vi "NovaParts.vi"() -> ()   [LabVIEW 2012]
uses:
  <vilib>/addons/database/Connection.llb/DB Tools Open Connec (Path).vi
  <vilib>/addons/database/Connection.llb/Conn Execute.vi
  <vilib>/addons/database/Recordset.llb/Rec Fetch Recordset Data (R).vi
  <vilib>/addons/database/Recordset.llb/Rec Destroy - Connection.vi
  <vilib>/Utility/file.llb/Write To Spreadsheet File (string).vi
  <vilib>/addons/database/_DB Variant To Data/Database Variant To Data.xnode
  <vilib>/addons/database/NI_Database_API.lvlib
panel:
  out "error out":errorcluster
  out "Array 2":string[][](array[string])
  out "spreadsheet string":string
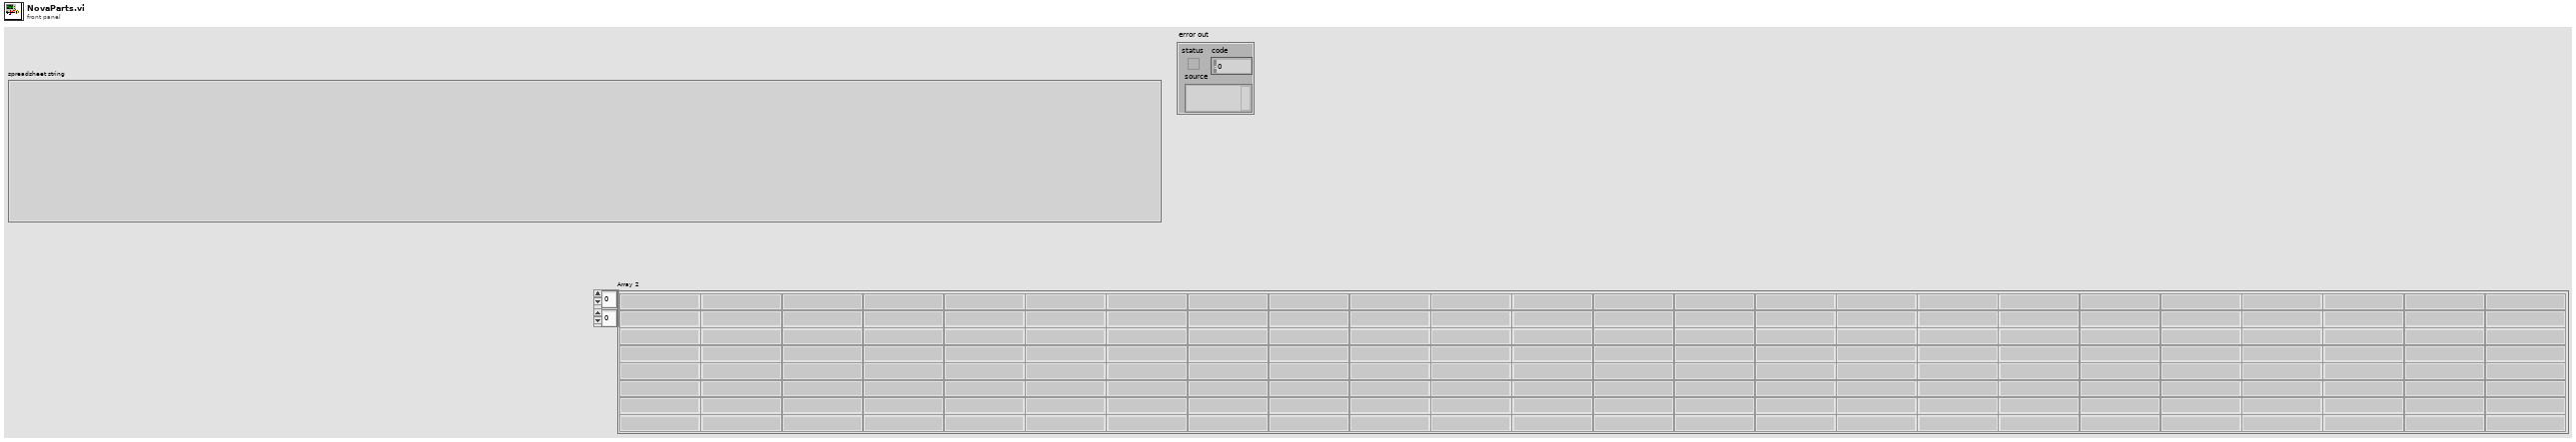
[diagram p1: front panel]
types:
  T1 = typedef "NI_Database_API.lvlib/Conn ObjectReference.ctl" = refnum<k1>
  T2 = typedef "NI_Database_API.lvlib/Rec ObjectReference.ctl" = refnum<k1>
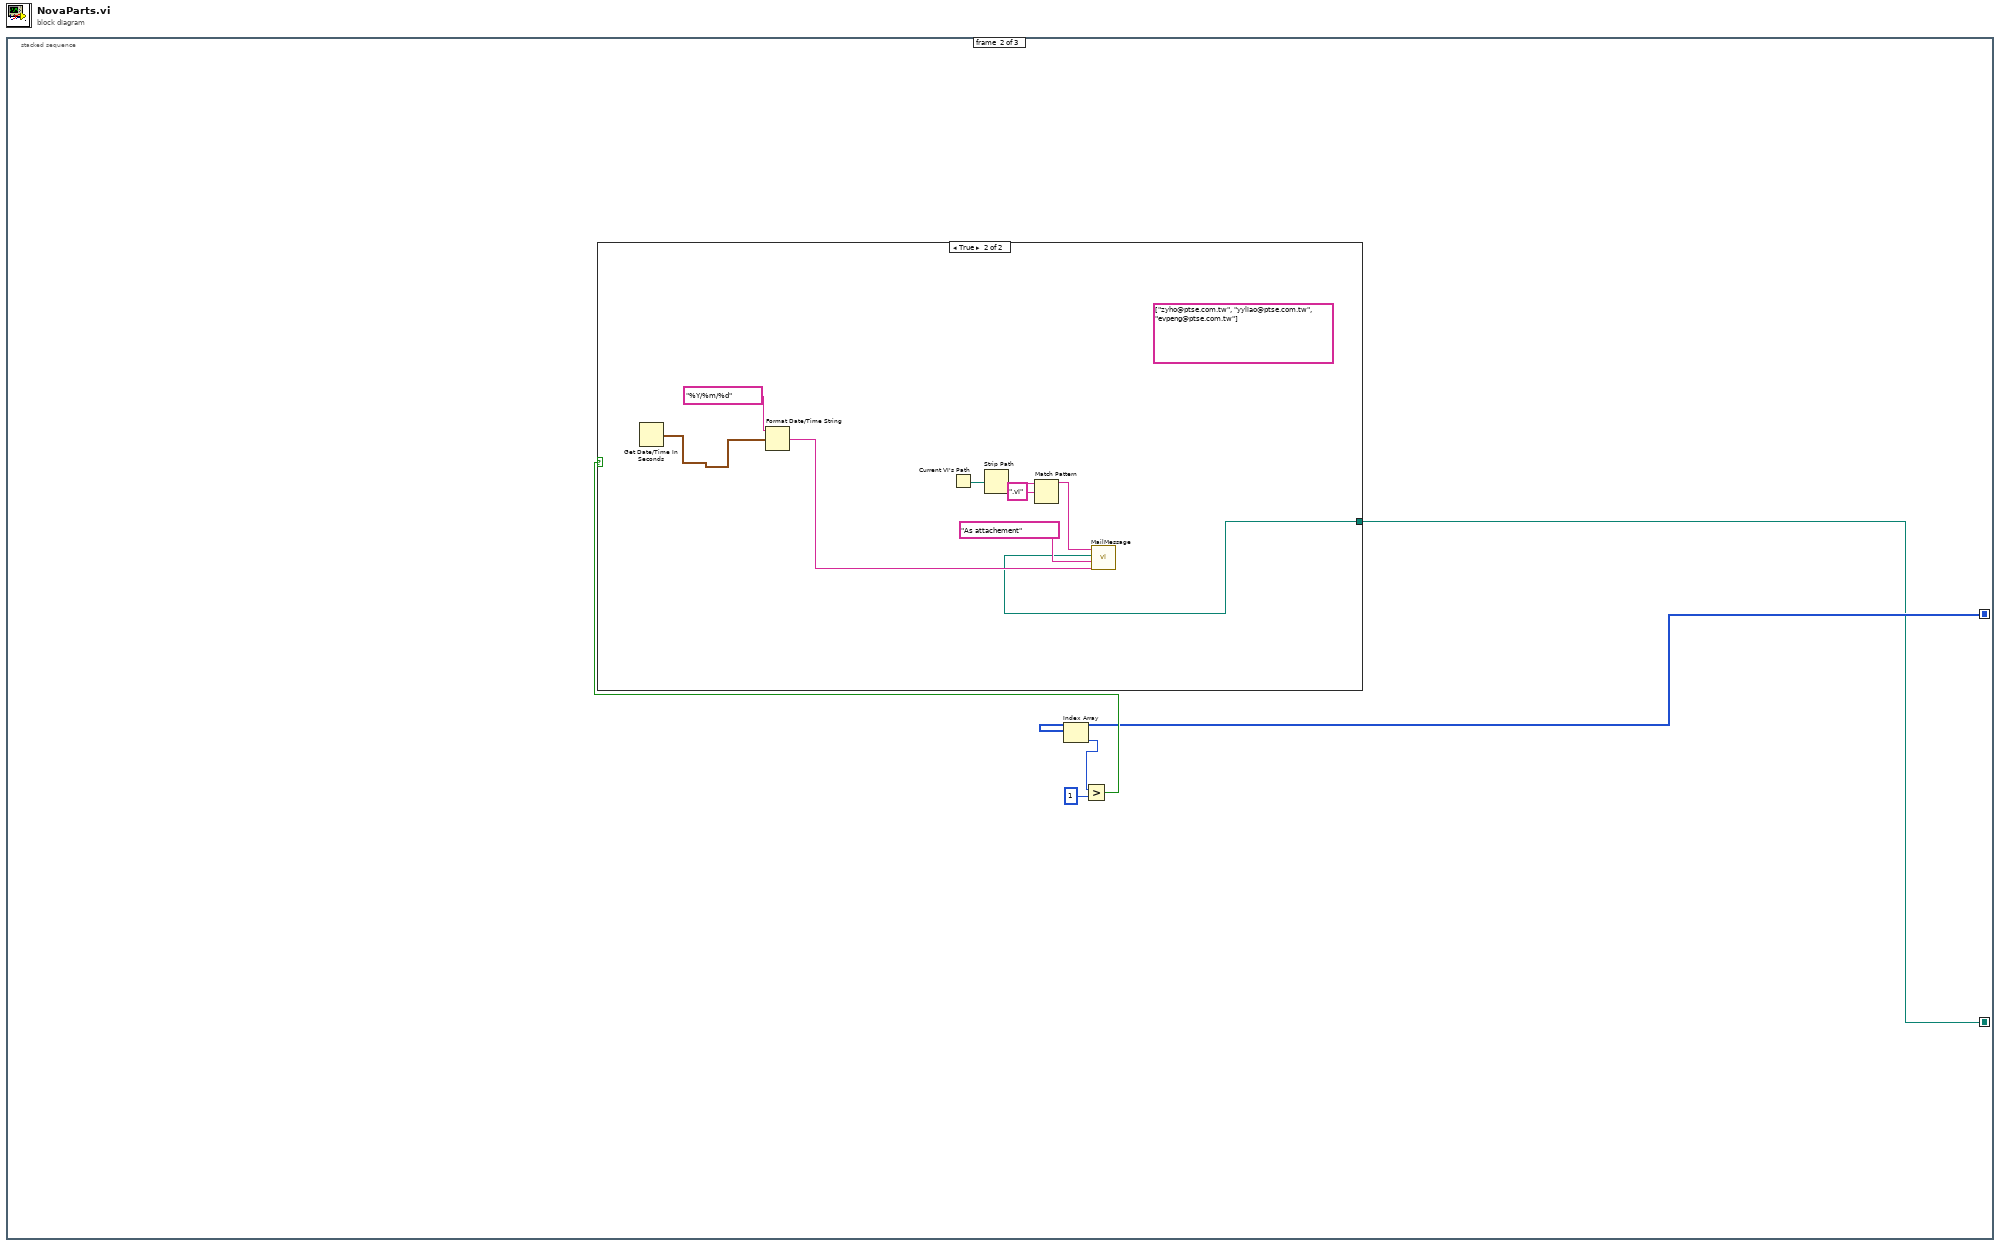
[diagram p0: block diagram]
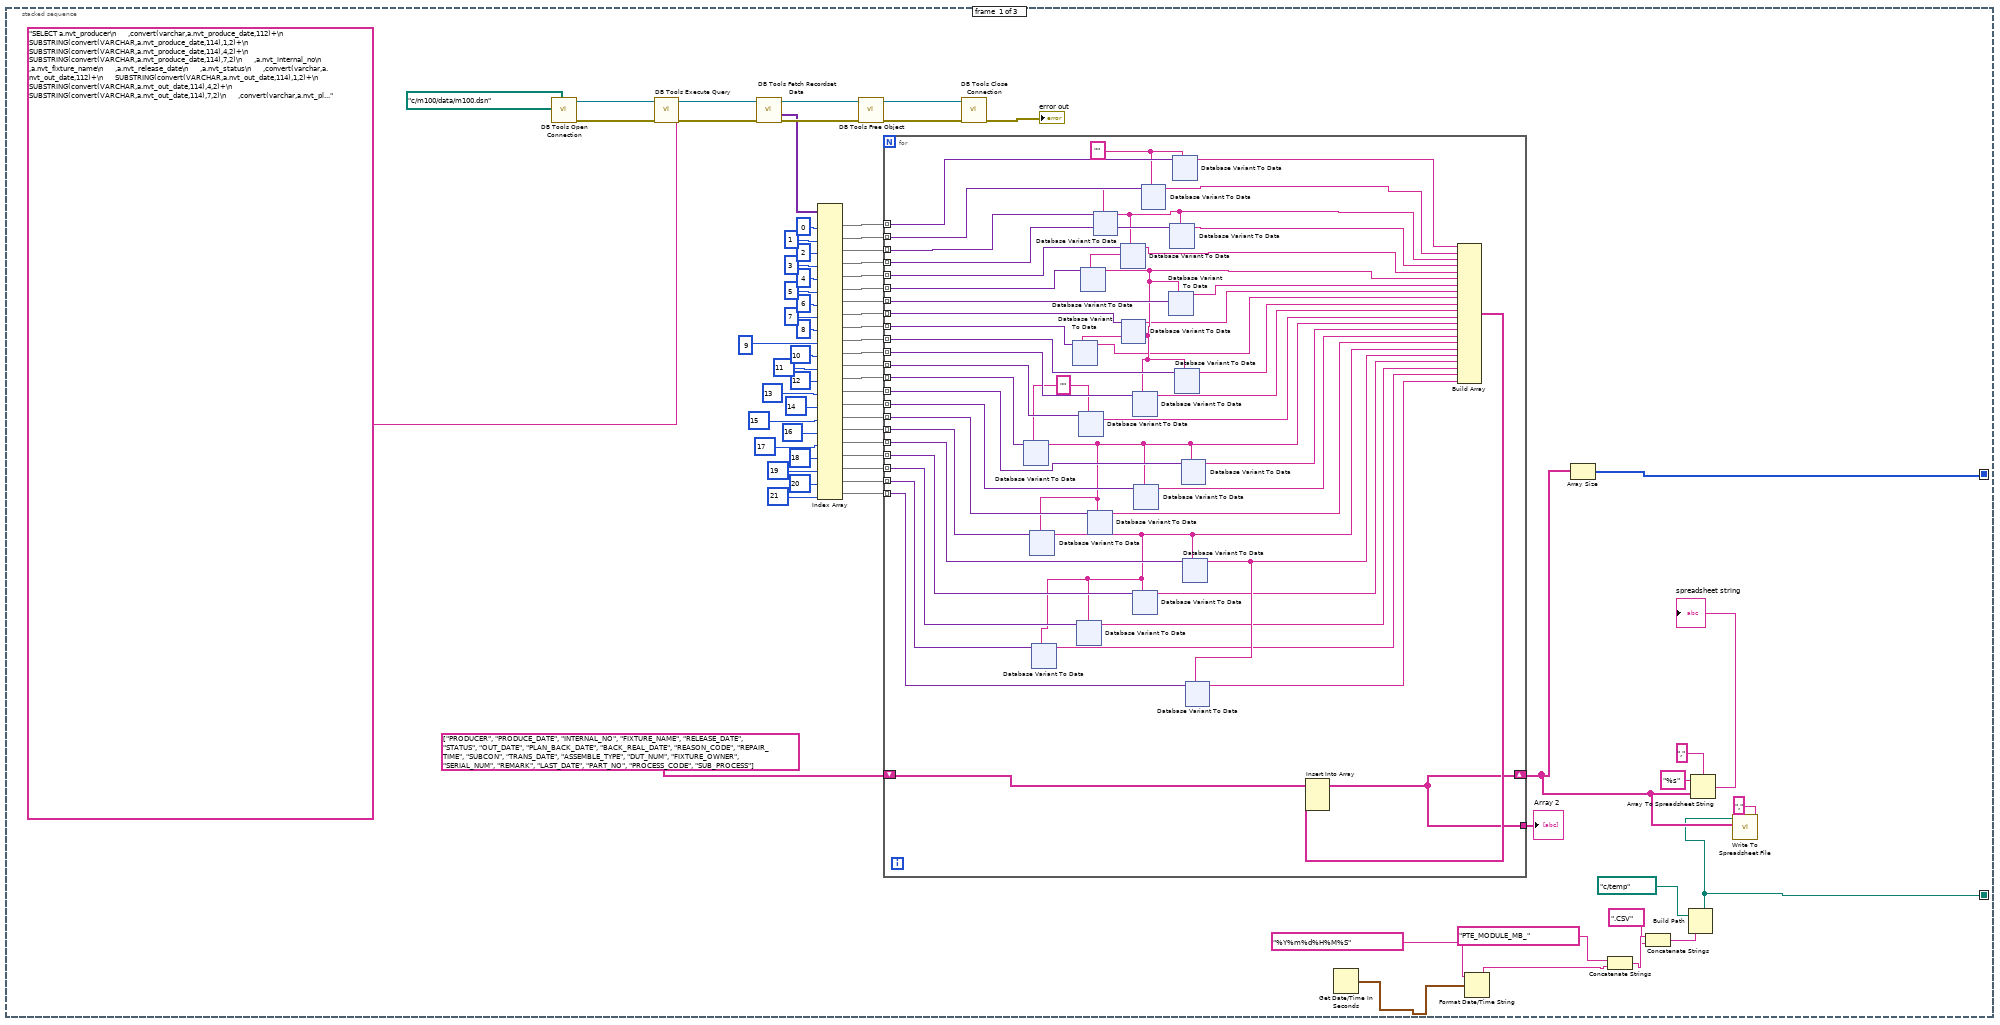
[diagram p2: hidden frame]
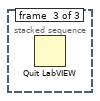
[diagram p4: hidden frame]
diagram:
  n1 = stacked-sequence {
    seq-local: [w41 _ _] -> [_ w828 _]
    seq-local: [w11 _ _] -> [_ w827 _]
    frame #0 {
      n2 = call-poly <vilib>:"DB Tools Open Connection.vi"("connection information"=path "c:/m100/data/m100.dsn") -> ("error out"=w68:errorcluster, "connection reference"=w72:T1)  [unwired: 7 in]
      n3 = call-poly <vilib>:"DB Tools Execute Query.vi"("error in (no error)"=w68, "SQL query"="SELECT a.nvt_producer\n      ,convert(varchar,a.nvt_produce_date,112)+\n      SUBSTRING(convert(VARCHAR,a.nvt_produce_date,114),1,2)+\n      SUBSTRING(convert(VARCHAR,a.nvt_produce_date,114),4,2)+\n      SUBSTRING(convert(VARCHAR,a.nvt_produce_date,114),7,2)\n      ,a.nvt_internal_no\n      ,a.nvt_fixture_name\n      ,a.nvt_release_date\n      ,a.nvt_status\n      ,convert(varchar,a.nvt_out_date,112)+\n      SUBSTRING(convert(VARCHAR,a.nvt_out_date,114),1,2)+\n      SUBSTRING(convert(VARCHAR,a.nvt_out_date,114),4,2)+\n      SUBSTRING(convert(VARCHAR,a.nvt_out_date,114),7,2)\n      ,convert(varchar,a.nvt_plan_back_date,112)+\n      SUBSTRING(convert(VARCHAR,a.nvt_plan_back_date,114),1,2)+\n      SUBSTRING(convert(VARCHAR,a.nvt_plan_back_date,114),4,2)+\n      SUBSTRING(convert(VARCHAR,a.nvt_plan_back_date,114),7,2)\n      ,convert(varchar,a.nvt_back_real_date,112)+\n      SUBSTRING(convert(VARCHAR,a.nvt_back_real_date,114),1,2)+\n      SUBSTRING(convert(VARCHAR,a.nvt_back_real_date,114),4,2)+\n      SUBSTRING(convert(VARCHAR,a.nvt_back_real_date,114),7,2)\n      ,a.nvt_reason_code\n      ,a.nvt_repair_time\n      ,a.nvt_subcon\n      ,convert(varchar,a.nvt_trans_date,112)+\n      SUBSTRING(convert(VARCHAR,a.nvt_trans_date,114),1,2)+\n      SUBSTRING(convert(VARCHAR,a.nvt_trans_date,114),4,2)+\n      SUBSTRING(convert(VARCHAR,a.nvt_trans_date,114),7,2)\n      ,a.nvt_assemble_type\n      ,a.nvt_dut_num\n      ,a.nvt_fixture_owner\n      ,a.nvt_serial_num\n      ,a.nvt_remark\n      ,convert(varchar,a.nvt_last_date,112)+\n      SUBSTRING(convert(VARCHAR,a.nvt_last_date,114),1,2)+\n      SUBSTRING(convert(VARCHAR,a.nvt_last_date,114),4,2)+\n      SUBSTRING(convert(VARCHAR,a.nvt_last_date,114),7,2)\n      ,a.nvt_part_no\n      ,a.nvt_process_code\n      ,a.nvt_sub_process\n from m100.dbo.nvt_parts a", "connection reference"=w72) -> ("error out"=w67:errorcluster, "recordset reference"=w71:T2)  [unwired: 5 in]
      n4 = call-poly <vilib>:"DB Tools Fetch Recordset Data.vi"("error in (no error)"=w67, "recordset reference"=w71) -> ("error out"=w66:errorcluster, "recordset data"=w35:variant[][], "recordset reference out"=w70:T2)  [unwired: 3 in]
      n5 = Index Array(array=w35, index (col) #1=0 ("disabled index (col)"), index (col) #2=1 ("index (col)"), index (col) #3=2 ("index (col)"), index (col) #4=3 ("index (col)"), index (col) #5=4 ("index (col)"), index (col) #6=5 ("index (col)"), index (col) #7=6 ("index (col)"), index (col) #8=7 ("index (col)"), index (col) #9=8 ("index (col)"), index (col) #10=9 ("index (col)"), index (col) #11=10 ("index (col)"), index (col) #12=11 ("index (col)"), index (col) #13=12 ("index (col)"), index (col) #14=13 ("index (col)"), index (col) #15=14 ("index (col)"), index (col) #16=15 ("index (col)"), index (col) #17=16 ("index (col)"), index (col) #18=17 ("index (col)"), index (col) #19=18 ("index (col)"), index (col) #20=19 ("index (col)"), index (col) #21=20 ("index (col)"), index (col) #22=21 ("index (col)")) -> (element #1=w52:variant[], element #2=w51:variant[], element #3=w50:variant[], element #4=w49:variant[], element #5=w48:variant[], element #6=w47:variant[], element #7=w46:variant[], element #8=w45:variant[], element #9=w44:variant[], element #10=w43:variant[], element #11=w42:variant[], element #12=w38:variant[], element #13=w37:variant[], element #14=w29:variant[], element #15=w28:variant[], element #16=w27:variant[], element #17=w26:variant[], element #18=w25:variant[], element #19=w4:variant[], element #20=w3:variant[], element #21=w2:variant[], element #22=w1:variant[])  [unwired: 22 in]
      n6 = call-poly <vilib>:"DB Tools Free Object.vi"("error in (no error)"=w66, "recordset reference"=w70) -> ("error out"=w65:errorcluster, "connection reference"=w69:T1)  [unwired: 8 in]
      n7 = for {
        tunnel: w52 -> [w122] mode=indexing
        tunnel: w51 -> [w121] mode=indexing
        tunnel: w50 -> [w120] mode=indexing
        tunnel: w49 -> [w119] mode=indexing
        tunnel: w48 -> [w118] mode=indexing
        tunnel: w47 -> [w117] mode=indexing
        tunnel: w46 -> [w116] mode=indexing
        tunnel: w45 -> [w115] mode=indexing
        tunnel: w44 -> [w114] mode=indexing
        tunnel: w43 -> [w113] mode=indexing
        tunnel: w42 -> [w112] mode=indexing
        tunnel: [w109] -> w24
        shift-right: [w109] -> w20
        shift-left: string[][] [["PRODUCER", "PRODUCE_DATE", "INTERNAL_NO", "FIXTURE_NAME", "RELEASE_DATE", "STATUS", "OUT_DATE", "PLAN_BACK_DATE", "BACK_REAL_DATE", "REASON_CODE", "REPAIR_TIME", "SUBCON", "TRANS_DATE", "ASSEMBLE_TYPE", "DUT_NUM", "FIXTURE_OWNER", "SERIAL_NUM", "REMARK", "LAST_DATE", "PART_NO", "PROCESS_CODE", "SUB_PROCESS"]] ("Array") -> [w108]
        tunnel: w38 -> [w107] mode=indexing
        tunnel: w37 -> [w106] mode=indexing
        tunnel: w29 -> [w92] mode=indexing
        tunnel: w28 -> [w91] mode=indexing
        tunnel: w27 -> [w90] mode=indexing
        tunnel: w26 -> [w89] mode=indexing
        tunnel: w25 -> [w88] mode=indexing
        tunnel: w4 -> [w83] mode=indexing
        tunnel: w3 -> [w82] mode=indexing
        tunnel: w2 -> [w81] mode=indexing
        tunnel: w1 -> [w80] mode=indexing
        w105 = ""
        w102 = ""
        n8 = xnode "Database Variant To Data"("database variant"=w106, "type"=w105) -> ("data"=w87:string)  [unwired: 1 in, 1 out]
        n9 = xnode "Database Variant To Data"("database variant"=w89, "type"=w87) -> ("data"=w79:string)  [unwired: 1 in, 1 out]
        n10 = xnode "Database Variant To Data"("database variant"=w81, "type"=w79) -> ("data"=w75:string)  [unwired: 1 in, 1 out]
        n11 = xnode "Database Variant To Data"("database variant"=w82, "type"=w79) -> ("data"=w76:string)  [unwired: 1 in, 1 out]
        n12 = xnode "Database Variant To Data"("database variant"=w107, "type"=w105) -> ("data"=w104:string)  [unwired: 1 in, 1 out]
        n13 = xnode "Database Variant To Data"("database variant"=w90, "type"=w87) -> ("data"=w84:string)  [unwired: 1 in, 1 out]
        n14 = xnode "Database Variant To Data"("database variant"=w120, "type"=w102) -> ("data"=w99:string)  [unwired: 1 in, 1 out]
        n15 = xnode "Database Variant To Data"("database variant"=w117, "type"=w99) -> ("data"=w98:string)  [unwired: 1 in, 1 out]
        n16 = xnode "Database Variant To Data"("database variant"=w114, "type"=w98) -> ("data"=w95:string)  [unwired: 1 in, 1 out]
        n17 = xnode "Database Variant To Data"("database variant"=w118, "type"=w99) -> ("data"=w100:string)  [unwired: 1 in, 1 out]
        n18 = xnode "Database Variant To Data"("database variant"=w115, "type"=w98) -> ("data"=w96:string)  [unwired: 1 in, 1 out]
        n19 = xnode "Database Variant To Data"("database variant"=w112, "type"=w98) -> ("data"=w93:string)  [unwired: 1 in, 1 out]
        n20 = xnode "Database Variant To Data"("database variant"=w83, "type"=w79) -> ("data"=w77:string)  [unwired: 1 in, 1 out]
        n21 = xnode "Database Variant To Data"("database variant"=w91, "type"=w87) -> ("data"=w85:string)  [unwired: 1 in, 1 out]
        n22 = xnode "Database Variant To Data"("database variant"=w121, "type"=w102) -> ("data"=w103:string)  [unwired: 1 in, 1 out]
        n23 = xnode "Database Variant To Data"("database variant"=w116, "type"=w98) -> ("data"=w97:string)  [unwired: 1 in, 1 out]
        n24 = xnode "Database Variant To Data"("database variant"=w119, "type"=w99) -> ("data"=w101:string)  [unwired: 1 in, 1 out]
        n25 = xnode "Database Variant To Data"("database variant"=w122, "type"=w102) -> ("data"=w111:string)  [unwired: 1 in, 1 out]
        n26 = xnode "Database Variant To Data"("database variant"=w113, "type"=w98) -> ("data"=w94:string)  [unwired: 1 in, 1 out]
        n27 = xnode "Database Variant To Data"("database variant"=w92, "type"=w87) -> ("data"=w86:string)  [unwired: 1 in, 1 out]
        n28 = xnode "Database Variant To Data"("database variant"=w88, "type"=w79) -> ("data"=w78:string)  [unwired: 1 in, 1 out]
        n29 = xnode "Database Variant To Data"("database variant"=w80, "type"=w78) -> ("data"=w74:string)  [unwired: 1 in, 1 out]
        n30 = Build Array(w111, w103, w99, w101, w100, w98, w97, w96, w95, w94, w93, w104, w87, w86, w85, w84, w79, w78, w77, w76, w75, w74) -> (w110:string[])
        n31 = Insert Into Array(array=w108, new element=w110) -> (w109:string[][])  [unwired: 2 in]
      }
      "Array 2" <- w24
      n32 = call <vilib>:"DB Tools Close Connection.vi"("error in (no error)"=w65, "connection reference"=w69) -> ("error out"=→"error out":errorcluster)  [unwired: 5 in]
      n33 = Get Date/Time In Seconds() -> (seconds since 1Jan1904=w9:timestamp)
      n34 = Format Date/Time String(time format string (%c)="%Y%m%d%H%M%S", seconds (now)=w9) -> (date/time string=w12:string)  [unwired: 1 in]
      n35 = Array Size(array=w20) -> (size(s)=w41:i32[])
      n36 = Concatenate Strings("PTE_MODULE_MB_" ("string"), w12) -> (w16:string)
      n37 = Concatenate Strings(w16, ".CSV" ("string")) -> (w14:string)
      n38 = Build Path(base path=path "c:/temp", name or relative path=w14) -> (appended path=w11:path)
      n39 = Array To Spreadsheet String(delimiter (Tab)=",", array=w20, 3:"%s" ("format string")) -> (spreadsheet string=→"spreadsheet string":string)
      n40 = call-poly <vilib>:"Write To Spreadsheet File.vi"("delimiter (\\t)"="," ("delimiter (\\t)"), "2D data"=w20, "file path (dialog if empty)"=w11) -> ()  [unwired: 5 in, 1 out]
    }
    frame #1 {
      n41 = Index Array(array=w828) -> (element=w831:i32)  [unwired: 1 in]
      n42 = Greater?(x=w831, y=1) -> (0:w829:bool)
      n43 = case shown="True" w829 {
        tunnel: w827 -> [_ w832]
        frame False {
        }
        frame True {
          (unwired) string[] ["zyho@ptse.com.tw", "yyliao@ptse.com.tw", "evpeng@ptse.com.tw"] ("recipients")
          n44 = Get Date/Time In Seconds() -> (seconds since 1Jan1904=w839:timestamp)
          n45 = Format Date/Time String(time format string (%c)="%Y/%m/%d", seconds (now)=w839) -> (date/time string=w833:string)  [unwired: 1 in]
          n46 = Current VI's Path() -> (path=w838:path)
          n47 = Strip Path(path=w838) -> (name=w837:string)  [unwired: 1 out]
          n48 = Match Pattern(string=w837, regular expression=".vi") -> (before substring=w835:string)  [unwired: 1 in, 3 out]
          n49 = call "MailMessage.vi"("AddSubject"=w833, "message"="As attachement", "file path"=w832, "program"=w835) -> ()  [unwired: 8 in]
        }
      }
    }
    frame #2 {
      n50 = Quit LabVIEW() -> ()  [unwired: 1 in]
    }
  }
